vi "Do.vi"(8 "error in (no error)":errorcluster, 10 "Actor in":refnum<class "Actor.lvclass">, 11 "Analog Input Waveform Data Msg":refnum<class "Analog Input Waveform Data Msg.lvclass">) -> (0 "error out":errorcluster, 2 "Actor out":refnum<class "Actor.lvclass">)   [LabVIEW 2024, in "Root Tester.lvlib" / "Analog Input Waveform Data Msg.lvclass"]
doc: "This VI delivers the message to the actor by calling the appropriate method(s) on the actor."
uses:
  Analog Input Waveform Data Msg.lvclass
  <vilib>/ActorFramework/Actor/Actor.lvclass
  Root Tester/Root Tester.lvclass
  C:/Program Files (x86)/National Instruments/LabVIEW 2024/vi.lib/ActorFramework/Actor/Actor.lvclass
  34700b1e-4b1b-4205-ab4b-28631ba2a4c6.vi
  Analog Input Waveform Data Msg.lvclass/Analog Input Waveform Data Msg.ctl
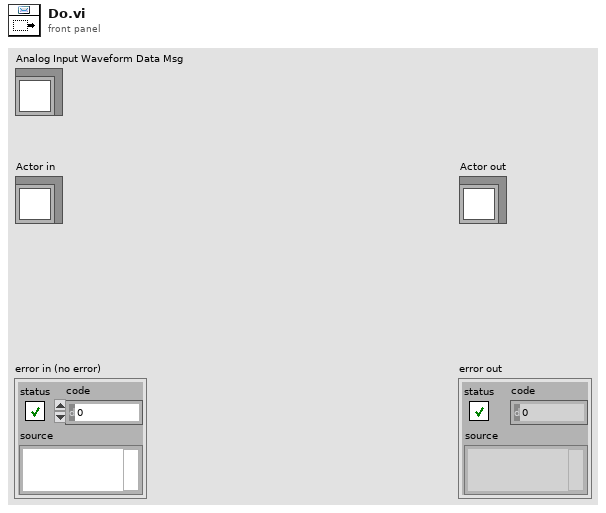
[diagram p1: front panel]
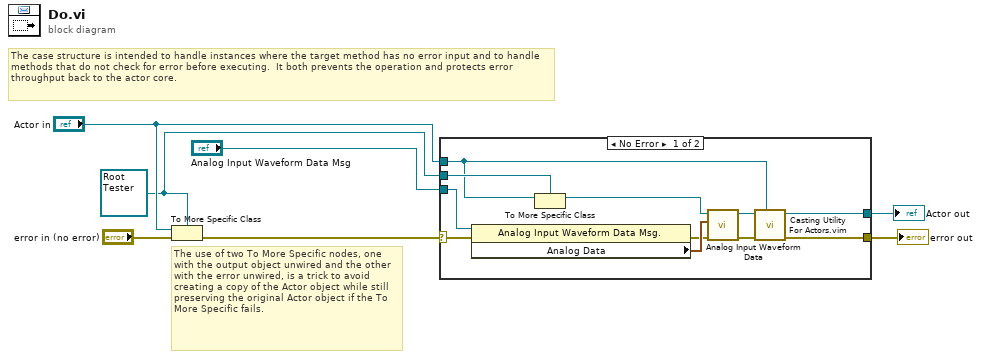
[diagram p0: block diagram]
diagram:
  w2 = refnum<class "Root Tester.lvclass"> refnum ("Actor in")
  # "The use of two To More Specific nodes, one with the output object unwired and the other with the error unwired, is a trick to avoid creating a copy of the Actor object while still preserving the original Actor object if the To More Specific fails."
  # "The case structure is intended to handle instances where the target method has no error input and to handle methods that do not check for error before executing.  It both prevents the operation and protects error throughput back to the actor core."
  n1 = To More Specific Class(target class=w2, reference="Actor in", error in="error in (no error)") -> (error out=w6:errorcluster)  [unwired: 1 out]
  n2 = case shown="No Error" w6 {
    selector: w6 -> [w9 w20]
    tunnel: [w13 w20] -> w5
    tunnel: [w12 w19] -> w4
    tunnel: "Actor in" -> [w16 w19]
    tunnel: w2 -> [w17 _]
    tunnel: "Analog Input Waveform Data Msg" -> [w11 _]
    frame No Error {
      n3 = property class="Analog Input Waveform Data Msg."(reference=w11, error in=w9) -> (error out=w8:errorcluster, "Analog Data"=w10:waveform(dbl)[])  [unwired: 1 out]
      n4 = To More Specific Class(target class=w17, reference=w16) -> (specific class reference=w18:refnum<class "Root Tester.lvclass">)  [unwired: 1 in, 1 out]
      n5 = call-dynamic "Analog Input Waveform Data.vi"("error in (no error)"=w8, "Analog Data"=w10, "Root Tester in"=w18) -> ("error out"=w14:errorcluster, "Root Tester out"=w15:refnum<class "Root Tester.lvclass">)  [unwired: 7 in]
      n6 = call "Casting Utility For Actors.vim"("type"=w16, "error in (no error)"=w14, "Actor in"=w15) -> ("error out"=w13:errorcluster, "Actor out"=w12:refnum<class "Actor.lvclass">)  [unwired: 7 in]
    }
    frame Error {
      # "If type check fails, pass the original object out again."
    }
  }
  "error out" <- w5
  "Actor out" <- w4
